vi "Format CSV.vi"(8 "error in (no error)":errorcluster, 9 "delimiter":string=",", 10 "CSV File Input":path, 11 "Original CSV Format":enum16{"Format A", "Format B"}(ring)) -> (0 "error out":errorcluster, 1 "Parcel Length":i32[](array[numeric]), 2 "All Terminal Data":T1(array[cluster]))   [LabVIEW 2017] (continued)
"48:51.9", "48:51.9", "48:51.9", "48:52.0", "48:52.0", "48:52.0", "48:52.1", "48:52.1", "48:52.1", "48:52.2", "48:52.2", "48:52.2", "48:52.3", "48:52.3", "48:52.3", "48:52.4", "48:52.4", "48:52.4", "48:52.5", "48:52.5", "48:52.5", "48:52.6", "48:52.6", "48:52.6", "48:52.7", "48:52.7", "48:52.7", "48:52.8", "48:52.8", "48:52.8", "48:52.9", "48:52.9", "48:52.9", "48:53.0", "48:53.0", "48:53.0", "48:53.1", "48:53.1", "48:53.1", "48:53.2", "48:53.2", "48:53.2", "48:53.3", "48:53.3", "48:53.3", "48:53.4", "48:53.4", "48:53.4", "48:53.5", "48:53.5", "48:53.5", "48:53.6", "48:53.6", "48:53.6", "48:53.7", "48:53.7", "48:53.7", "48:53.8", "48:53.8", "48:53.8", "48:53.9", "48:53.9", "48:53.9", "48:54.0", "48:54.0", "48:54.0", "48:54.1", "48:54.1", "48:54.1", "48:54.2", "48:54.2", "48:54.2", "48:54.3", "48:54.3", "48:54.3", "48:54.4", "48:54.4", "48:54.4", "48:54.5", "48:54.5", "48:54.5", "48:54.6", "48:54.6", "48:54.6", "48:54.7", "48:54.7", "48:54.7", "48:54.8", "48:54.8", "48:54.8", "48:54.9", "48:54.9", "48:54.9", "48:55.0", "48:55.0", "48:55.0", "48:55.1", "48:55.1", "48:55.1", "48:55.2", "48:55.2", "48:55.2", "48:55.3", "48:55.3", "48:55.3", "48:55.4", "48:55.4", "48:55.4", "48:55.5", "48:55.5", "48:55.5", "48:55.6", "48:55.6", "48:55.6", "48:55.7", "48:55.7", "48:55.7", "48:55.8", "48:55.8", "48:55.8", "48:55.9", "48:55.9", "48:55.9", "48:56.0", "48:56.0", "48:56.0", "48:56.1", "48:56.1", "48:56.1", "48:56.2", "48:56.2", "48:56.2", "48:56.3", "48:56.3", "48:56.3", "48:56.4", "48:56.4", "48:56.4", "48:56.5", "48:56.5", "48:56.5", "48:56.6", "48:56.6", "48:56.6", "48:56.7", "48:56.7", "48:56.7", "48:56.8", "48:56.8", "48:56.8", "48:56.9", "48:56.9", "48:56.9", "48:57.0", "48:57.0", "48:57.0", "48:57.1", "48:57.1", "48:57.1", "48:57.2", "48:57.2", "48:57.2", "48:57.3", "48:57.3", "48:57.3", "48:57.4", "48:57.4", "48:57.4", "48:57.5", "48:57.5", "48:57.5", "48:57.6", "48:57.6", "48:57.6", "48:57.7", "48:57.7", "48:57.7", "48:57.8", "48:57.8", "48:57.8", "48:57.9", "48:57.9", "48:57.9", "48:58.0", "48:58.0", "48:58.0", "48:58.1", "48:58.1", "48:58.1", "48:58.2", "48:58.2", "48:58.2", "48:58.3", "48:58.3", "48:58.3", "48:58.4", "48:58.4", "48:58.4", "48:58.5", "48:58.5", "48:58.5", "48:58.6", "48:58.6", "48:58.6", "48:58.7", "48:58.7", "48:58.7", "48:58.8", "48:58.8", "48:58.8", "48:58.9", "48:58.9", "48:58.9", "48:59.0", "48:59.0", "48:59.0", "48:59.1", "48:59.1", "48:59.1", "48:59.2", "48:59.2", "48:59.2", "48:59.3", "48:59.3", "48:59.3", "48:59.4", "48:59.4", "48:59.4", "48:59.5", "48:59.5", "48:59.5", "48:59.6", "48:59.6", "48:59.6", "48:59.7", "48:59.7", "48:59.7", "48:59.8", "48:59.8", "48:59.8", "48:59.9", "48:59.9", "48:59.9", "49:00.0", "49:00.0", "49:00.0", "49:00.1", "49:00.1", "49:00.1", "49:00.2", "49:00.2", "49:00.2", "49:00.3", "49:00.3", "49:00.3", "49:00.4", "49:00.4", "49:00.4", "49:00.5", "49:00.5", "49:00.5", "49:00.6", "49:00.6", "49:00.6", "49:00.7", "49:00.7", "49:00.7", "49:00.8", "49:00.8", "49:00.8", "49:00.9", "49:00.9", "49:00.9", "49:01.0", "49:01.0", "49:01.0", "49:01.1", "49:01.1", "49:01.1", "49:01.2", "49:01.2", "49:01.2", "49:01.3", "49:01.3", "49:01.3", "49:01.4", "49:01.4", "49:01.4", "49:01.5", "49:01.5", "49:01.5", "49:01.6", "49:01.6", "49:01.6", "49:01.7", "49:01.7", "49:01.7", "49:01.8", "49:01.8", "49:01.8", "49:01.9", "49:01.9", "49:01.9", "49:02.0", "49:02.0", "49:02.0", "49:02.1", "49:02.1", "49:02.1", "49:02.2", "49:02.2", "49:02.2", "49:02.3", "49:02.3", "49:02.3", "49:02.4", "49:02.4", "49:02.4", "49:02.5", "49:02.5", "49:02.5", "49:02.6", "49:02.6", "49:02.6", "49:02.7", "49:02.7", "49:02.7", "49:02.8", "49:02.8", "49:02.8", "49:02.9", "49:02.9", "49:02.9", "49:03.0", "49:03.0", "49:03.0", "49:03.1", "49:03.1", "49:03.1", "49:03.2", "49:03.2", "49:03.2", "49:03.3", "49:03.3", "49:03.3", "49:03.4", "49:03.4", "49:03.4", "49:03.5", "49:03.5", "49:03.5", "49:03.6", "49:03.6", "49:03.6", "49:03.7", "49:03.7", "49:03.7", "49:03.8", "49:03.8", "49:03.8", "49:03.9", "49:03.9", "49:03.9", "49:04.0", "49:04.0", "49:04.0", "49:04.1", "49:04.1", "49:04.1", "49:04.2", "49:04.2", "49:04.2", "49:04.3", "49:04.3", "49:04.3", "49:04.4", "49:04.4", "49:04.4", "49:04.5", "49:04.5", "49:04.5", "49:04.6", "49:04.6", "49:04.6", "49:04.7", "49:04.7", "49:04.7", "49:04.8", "49:04.8", "49:04.8", "49:04.9", "49:04.9", "49:04.9", "49:05.0", "49:05.0", "49:05.0", "49:05.1", "49:05.1", "49:05.1", "49:05.2", "49:05.2", "49:05.2", "49:05.3", "49:05.3", "49:05.3", "49:05.4", "49:05.4", "49:05.4", "49:05.5", "49:05.5", "49:05.5", "49:05.6", "49:05.6", "49:05.6", "49:05.7", "49:05.7", "49:05.7", "49:05.8", "49:05.8", "49:05.8", "49:05.9", "49:05.9", "49:05.9", "49:06.0", "49:06.0", "49:06.0", "49:06.1", "49:06.1", "49:06.1", "49:06.2", "49:06.2", "49:06.2", "49:06.3", "49:06.3", "49:06.3", "49:06.4", "49:06.4", "49:06.4", "49:06.5", "49:06.5", "49:06.5", "49:06.6", "49:06.6", "49:06.6", "49:06.7", "49:06.7", "49:06.7", "49:06.8", "49:06.8", "49:06.8", "49:06.9", "49:06.9", "49:06.9", "49:07.0", "49:07.0", "49:07.0", "49:07.1", "49:07.1", "49:07.1", "49:07.2", "49:07.2", "49:07.2", "49:07.3", "49:07.3", "49:07.3", "49:07.4", "49:07.4", "49:07.4", "49:07.5", "49:07.5", "49:07.5", "49:07.6", "49:07.6", "49:07.6", "49:07.7", "49:07.7", "49:07.7", "49:07.8", "49:07.8", "49:07.8", "49:07.9", "49:07.9", "49:07.9", "49:08.0", "49:08.0", "49:08.0", "49:08.1", "49:08.1", "49:08.1", "49:08.2", "49:08.2", "49:08.2", "49:08.3", "49:08.3", "49:08.3", "49:08.4", "49:08.4", "49:08.4", "49:08.5", "49:08.5", "49:08.5", "49:08.6", "49:08.6", "49:08.6", "49:08.7", "49:08.7", "49:08.7", "49:08.8", "49:08.8", "49:08.8", "49:08.9", "49:08.9", "49:08.9", "49:09.0", "49:09.0", "49:09.0", "49:09.1", "49:09.1", "49:09.1", "49:09.2", "49:09.2", "49:09.2", "49:09.3", "49:09.3", "49:09.3", "49:09.4", "49:09.4", "49:09.4", "49:09.5", "49:09.5", "49:09.5", "49:09.6", "49:09.6", "49:09.6", "49:09.7", "49:09.7", "49:09.7", "49:09.8", "49:09.8", "49:09.8", "49:09.9", "49:09.9", "49:09.9", "49:10.0", "49:10.0", "49:10.0", "49:10.1", "49:10.1", "49:10.1", "49:10.2", "49:10.2", "49:10.2", "49:10.3", "49:10.3", "49:10.3", "49:10.4", "49:10.4", "49:10.4", "49:10.5", "49:10.5", "49:10.5", "49:10.6", "49:10.6", "49:10.6", "49:10.7", "49:10.7", "49:10.7", "49:10.8", "49:10.8", "49:10.8", "49:10.9", "49:10.9", "49:10.9", "49:11.0", "49:11.0", "49:11.0", "49:11.1", "49:11.1", "49:11.1", "49:11.2", "49:11.2", "49:11.2", "49:11.3", "49:11.3", "49:11.3", "49:11.4", "49:11.4", "49:11.4", "49:11.5", "49:11.5", "49:11.5", "49:11.6", "49:11.6", "49:11.6", "49:11.7", "49:11.7", "49:11.7", "49:11.8", "49:11.8", "49:11.8", "49:11.9", "49:11.9", "49:11.9", "49:12.0", "49:12.0", "49:12.0", "49:12.1", "49:12.1", "49:12.1", "49:12.2", "49:12.2", "49:12.2", "49:12.3", "49:12.3", "49:12.3", "49:12.4", "49:12.4", "49:12.4", "49:12.5", "49:12.5", "49:12.5", "49:12.6", "49:12.6", "49:12.6", "49:12.7", "49:12.7", "49:12.7", "49:12.8", "49:12.8", "49:12.8", "49:12.9", "49:12.9", "49:12.9", "49:13.0", "49:13.0", "49:13.0", "49:13.1", "49:13.1", "49:13.1", "49:13.2", "49:13.2", "49:13.2", "49:13.3", "49:13.3", "49:13.3", "49:13.4", "49:13.4", "49:13.4", "49:13.5", "49:13.5", "49:13.5", "49:13.6", "49:13.6", "49:13.6", "49:13.7", "49:13.7", "49:13.7", "49:13.8", "49:13.8", "49:13.8", "49:13.9", "49:13.9", "49:13.9", "49:14.0", "49:14.0", "49:14.0", "49:14.1", "49:14.1", "49:14.1", "49:14.2", "49:14.2", "49:14.2", "49:14.3", "49:14.3", "49:14.3", "49:14.4", "49:14.4", "49:14.4", "49:14.5", "49:14.5", "49:14.5", "49:14.6", "49:14.6", "49:14.6", "49:14.7", "49:14.7", "49:14.7", "49:14.8", "49:14.8", "49:14.8", "49:14.9", "49:14.9", "49:14.9", "49:15.0", "49:15.0", "49:15.0", "49:15.1", "49:15.1", "49:15.1", "49:15.2", "49:15.2", "49:15.2", "49:15.3", "49:15.3", "49:15.3", "49:15.4", "49:15.4", "49:15.4", "49:15.5", "49:15.5", "49:15.5", "49:15.6", "49:15.6", "49:15.6", "49:15.7", "49:15.7", "49:15.7", "49:15.8", "49:15.8", "49:15.8", "49:15.9", "49:15.9", "49:15.9", "49:16.0", "49:16.0", "49:16.0", "49:16.1", "49:16.1", "49:16.1", "49:16.2", "49:16.2", "49:16.2", "49:16.3", "49:16.3", "49:16.3", "49:16.4", "49:16.4", "49:16.4", "49:16.5", "49:16.5", "49:16.5", "49:16.6", "49:16.6", "49:16.6", "49:16.7", "49:16.7", "49:16.7", "49:16.8", "49:16.8", "49:16.8", "49:16.9", "49:16.9", "49:16.9", "49:17.0", "49:17.0", "49:17.0", "49:17.1", "49:17.1", "49:17.1", "49:17.2", "49:17.2", "49:17.2", "49:17.3", "49:17.3", "49:17.3", "49:17.4", "49:17.4", "49:17.4", "49:17.5", "49:17.5", "49:17.5", "49:17.6", "49:17.6", "49:17.6", "49:17.7", "49:17.7", "49:17.7", "49:17.8", "49:17.8", "49:17.8", "49:17.9", "49:17.9", "49:17.9", "49:18.0", "49:18.0", "49:18.0", "49:18.1", "49:18.1", "49:18.1", "49:18.2", "49:18.2", "49:18.2", "49:18.3", "49:18.3", "49:18.3", "49:18.4", "49:18.4", "49:18.4", "49:18.5", "49:18.5", "49:18.5", "49:18.6", "49:18.6", "49:18.6", "49:18.7", "49:18.7", "49:18.7", "49:18.8", "49:18.8", "49:18.8", "49:18.9", "49:18.9", "49:18.9", "49:19.0", "49:19.0", "49:19.0", "49:19.1", "49:19.1", "49:19.1", "49:19.2", "49:19.2", "49:19.2", "49:19.3", "49:19.3", "49:19.3", "49:19.4", "49:19.4", "49:19.4", "49:19.5", "49:19.5", "49:19.5", "49:19.6", "49:19.6", "49:19.6", "49:19.7", "49:19.7", "49:19.7", "49:19.8", "49:19.8", "49:19.8", "49:19.9", "49:19.9", "49:19.9", "49:20.0", "49:20.0", "49:20.0", "49:20.1", "49:20.1", "49:20.1", "49:20.2", "49:20.2", "49:20.2", "49:20.3", "49:20.3", "49:20.3", "49:20.4", "49:20.4", "49:20.4", "49:20.5", "49:20.5", "49:20.5", "49:20.6", "49:20.6", "49:20.6", "49:20.7", "49:20.7", "49:20.7", "49:20.8", "49:20.8", "49:20.8", "49:20.9", "49:20.9", "49:20.9", "49:21.0", "49:21.0", "49:21.0", "49:21.1", "49:21.1", "49:21.1", "49:21.2", "49:21.2", "49:21.2", "49:21.3", "49:21.3", "49:21.3", "49:21.4", "49:21.4", "49:21.4", "49:21.5", "49:21.5", "49:21.5", "49:21.6", "49:21.6", "49:21.6", "49:21.7", "49:21.7", "49:21.7", "49:21.8", "49:21.8", "49:21.8", "49:21.9", "49:21.9", "49:21.9", "49:22.0", "49:22.0", "49:22.0", "49:22.1", "49:22.1", "49:22.1", "49:22.2", "49:22.2", "49:22.2", "49:22.3", "49:22.3", "49:22.3", "49:22.4", "49:22.4", "49:22.4", "49:22.5", "49:22.5", "49:22.5", "49:22.6", "49:22.6", "49:22.6", "49:22.7", "49:22.7", "49:22.7", "49:22.8", "49:22.8", "49:22.8", "49:22.9", "49:22.9", "49:22.9", "49:23.0", "49:23.0", "49:23.0", "49:23.1", "49:23.1", "49:23.1", "49:23.2", "49:23.2", "49:23.2", "49:23.3", "49:23.3", "49:23.3", "49:23.4", "49:23.4", "49:23.4", "49:23.5", "49:23.5", "49:23.5", "49:23.6", "49:23.6", "49:23.6", "49:23.7", "49:23.7", "49:23.7", "49:23.8", "49:23.8", "49:23.8", "49:23.9", "49:23.9", "49:23.9", "49:24.0", "49:24.0", "49:24.0", "49:24.1", "49:24.1", "49:24.1", "49:24.2", "49:24.2", "49:24.2", "49:24.3", "49:24.3", "49:24.3", "49:24.4", "49:24.4", "49:24.4", "49:24.5", "49:24.5", "49:24.5", "49:24.6", "49:24.6", "49:24.6", "49:24.7", "49:24.7", "49:24.7", "49:24.8", "49:24.8", "49:24.8", "49:24.9", "49:24.9", "49:24.9", "49:25.0", "49:25.0", "49:25.0", "49:25.1", "49:25.1", "49:25.1", "49:25.2", "49:25.2", "49:25.2", "49:25.3", "49:25.3", "49:25.3", "49:25.4", "49:25.4", "49:25.4", "49:25.5", "49:25.5", "49:25.5", "49:25.6", "49:25.6", "49:25.6", "49:25.7", "49:25.7", "49:25.7", "49:25.8", "49:25.8", "49:25.8", "49:25.9", "49:25.9", "49:25.9", "49:26.0", "49:26.0", "49:26.0", "49:26.1", "49:26.1", "49:26.1", "49:26.2", "49:26.2", "49:26.2", "49:26.3", "49:26.3", "49:26.3", "49:26.4", "49:26.4", "49:26.4", "49:26.5", "49:26.5", "49:26.5", "49:26.6", "49:26.6", "49:26.6", "49:26.7", "49:26.7", "49:26.7", "49:26.8", "49:26.8", "49:26.8", "49:26.9", "49:26.9", "49:26.9", "49:27.0", "49:27.0", "49:27.0", "49:27.1", "49:27.1", "49:27.1", "49:27.2", "49:27.2", "49:27.2", "49:27.3", "49:27.3", "49:27.3", "49:27.4", "49:27.4", "49:27.4", "49:27.5", "49:27.5", "49:27.5", "49:27.6", "49:27.6", "49:27.6", "49:27.7", "49:27.7", "49:27.7", "49:27.8", "49:27.8", "49:27.8", "49:27.9", "49:27.9", "49:27.9", "49:28.0", "49:28.0", "49:28.0", "49:28.1", "49:28.1", "49:28.1", "49:28.2", "49:28.2", "49:28.2", "49:28.3", "49:28.3", "49:28.3", "49:28.4", "49:28.4", "49:28.4", "49:28.5", "49:28.5", "49:28.5", "49:28.6", "49:28.6", "49:28.6", "49:28.7", "49:28.7", "49:28.7", "49:28.8", "49:28.8", "49:28.8", "49:28.9", "49:28.9", "49:28.9", "49:29.0", "49:29.0", "49:29.0", "49:29.1", "49:29.1", "49:29.1", "49:29.2", "49:29.2", "49:29.2", "49:29.3", "49:29.3", "49:29.3", "49:29.4", "49:29.4", "49:29.4", "49:29.5", "49:29.5", "49:29.5", "49:29.6", "49:29.6", "49:29.6", "49:29.7", "49:29.7", "49:29.7", "49:29.8", "49:29.8", "49:29.8", "49:29.9", "49:29.9", "49:29.9", "49:30.0", "49:30.0", "49:30.0", "49:30.1", "49:30.1", "49:30.1", "49:30.2", "49:30.2", "49:30.2", "49:30.3", "49:30.3", "49:30.3", "49:30.4", "49:30.4", "49:30.4", "49:30.5", "49:30.5", "49:30.5", "49:30.6", "49:30.6", "49:30.6", "49:30.7", "49:30.7", "49:30.7", "49:30.8", "49:30.8", "49:30.8", "49:30.9", "49:30.9", "49:30.9", "49:31.0", "49:31.0", "49:31.0", "49:31.1", "49:31.1", "49:31.1", "49:31.2", "49:31.2", "49:31.2", "49:31.3", "49:31.3", "49:31.3", "49:31.4", "49:31.4", "49:31.4", "49:31.5", "49:31.5", "49:31.5", "49:31.6", "49:31.6", "49:31.6", "49:31.7", "49:31.7", "49:31.7", "49:31.8", "49:31.8", "49:31.8", "49:31.9", "49:31.9", "49:31.9", "49:32.0", "49:32.0", "49:32.0", "49:32.1", "49:32.1", "49:32.1", "49:32.2", "49:32.2", "49:32.2", "49:32.3", "49:32.3", "49:32.3", "49:32.4", "49:32.4", "49:32.4", "49:32.5", "49:32.5", "49:32.5", "49:32.6", "49:32.6", "49:32.6", "49:32.7", "49:32.7", "49:32.7", "49:32.8", "49:32.8", "49:32.8", "49:32.9", "49:32.9", "49:32.9", "49:33.0", "49:33.0", "49:33.0", "49:33.1", "49:33.1", "49:33.1", "49:33.2", "49:33.2", "49:33.2", "49:33.3", "49:33.3", "49:33.3", "49:33.4", "49:33.4", "49:33.4", "49:33.5", "49:33.5", "49:33.5", "49:33.6", "49:33.6", "49:33.6", "49:33.7", "49:33.7", "49:33.7", "49:33.8", "49:33.8", "49:33.8", "49:33.9", "49:33.9", "49:33.9", "49:34.0", "49:34.0", "49:34.0", "49:34.1", "49:34.1", "49:34.1", "49:34.2", "49:34.2", "49:34.2", "49:34.3", "49:34.3", "49:34.3", "49:34.4", "49:34.4", "49:34.4", "49:34.5", "49:34.5", "49:34.5", "49:34.6", "49:34.6", "49:34.6", "49:34.7", "49:34.7", "49:34.7", "49:34.8", "49:34.8", "49:34.8", "49:34.9", "49:34.9", "49:34.9", "49:35.0", "49:35.0", "49:35.0", "49:35.1", "49:35.1", "49:35.1", "49:35.2", "49:35.2", "49:35.2", "49:35.3", "49:35.3", "49:35.3", "49:35.4", "49:35.4", "49:35.4", "49:35.5", "49:35.5", "49:35.5", "49:35.6", "49:35.6", "49:35.6", "49:35.7", "49:35.7", "49:35.7", "49:35.8", "49:35.8", "49:35.8", "49:35.9", "49:35.9", "49:35.9", "49:36.0", "49:36.0", "49:36.0", "49:36.1", "49:36.1", "49:36.1", "49:36.2", "49:36.2", "49:36.2", "49:36.3", "49:36.3", "49:36.3", "49:36.4", "49:36.4", "49:36.4", "49:36.5", "49:36.5", "49:36.5", "49:36.6", "49:36.6", "49:36.6", "49:36.7", "49:36.7", "49:36.7", "49:36.8", "49:36.8", "49:36.8", "49:36.9", "49:36.9", "49:36.9", "49:37.0", "49:37.0", "49:37.0", "49:37.1", "49:37.1", "49:37.1", "49:37.2", "49:37.2", "49:37.2", "49:37.3", "49:37.3", "49:37.3", "49:37.4", "49:37.4", "49:37.4", "49:37.5", "49:37.5", "49:37.5", "49:37.6", "49:37.6", "49:37.6", "49:37.7", "49:37.7", "49:37.7", "49:37.8", "49:37.8", "49:37.8", "49:37.9", "49:37.9", "49:37.9", "49:38.0", "49:38.0", "49:38.0", "49:38.1", "49:38.1", "49:38.1", "49:38.2", "49:38.2", "49:38.2", "49:38.3", "49:38.3", "49:38.3", "49:38.4", "49:38.4", "49:38.4", "49:38.5", "49:38.5", "49:38.5", "49:38.6", "49:38.6", "49:38.6", "49:38.7", "49:38.7", "49:38.7", "49:38.8", "49:38.8", "49:38.8", "49:38.9", "49:38.9", "49:38.9", "49:39.0", "49:39.0", "49:39.0", "49:39.1", "49:39.1", "49:39.1", "49:39.2", "49:39.2", "49:39.2", "49:39.3", "49:39.3", "49:39.3", "49:39.4", "49:39.4", "49:39.4", "49:39.5", "49:39.5", "49:39.5", "49:39.6", "49:39.6", "49:39.6", "49:39.7", "49:39.7", "49:39.7", "49:39.8", "49:39.8", "49:39.8", "49:39.9", "49:39.9", "49:39.9", "49:40.0", "49:40.0", "49:40.0", "49:40.1", "49:40.1", "49:40.1", "49:40.2", "49:40.2", "49:40.2", "49:40.3", "49:40.3", "49:40.3", "49:40.4", "49:40.4", "49:40.4", "49:40.5", "49:40.5", "49:40.5", "49:40.6", "49:40.6", "49:40.6", "49:40.7", "49:40.7", "49:40.7", "49:40.8", "49:40.8", "49:40.8", "49:40.9", "49:40.9", "49:40.9", "49:41.0", "49:41.0", "49:41.0", "49:41.1", "49:41.1", "49:41.1", "49:41.2", "49:41.2", "49:41.2", "49:41.3", "49:41.3", "49:41.3", "49:41.4", "49:41.4", "49:41.4", "49:41.5", "49:41.5", "49:41.5", "49:41.6", "49:41.6", "49:41.6", "49:41.7", "49:41.7", "49:41.7", "49:41.8", "49:41.8", "49:41.8", "49:41.9", "49:41.9", "49:41.9", "49:42.0", "49:42.0", "49:42.0", "49:42.1", "49:42.1", "49:42.1", "49:42.2", "49:42.2", "49:42.2", "49:42.3", "49:42.3", "49:42.3", "49:42.4", "49:42.4", "49:42.4", "49:42.5", "49:42.5", "49:42.5", "49:42.6", "49:42.6", "49:42.6", "49:42.7", "49:42.7", "49:42.7", "49:42.8", "49:42.8", "49:42.8", "49:42.9", "49:42.9", "49:42.9", "49:43.0", "49:43.0", "49:43.0", "49:43.1", "49:43.1", "49:43.1", "49:43.2", "49:43.2", "49:43.2", "49:43.3", "49:43.3", "49:43.3", "49:43.4", "49:43.4", "49:43.4", "49:43.5", "49:43.5", "49:43.5", "49:43.6", "49:43.6", "49:43.6", "49:43.7", "49:43.7", "49:43.7", "49:43.8", "49:43.8", "49:43.8", "49:43.9", "49:43.9", "49:43.9", "49:44.0", "49:44.0", "49:44.0", "49:44.1", "49:44.1", "49:44.1", "49:44.2", "49:44.2", "49:44.2", "49:44.3", "49:44.3", "49:44.3", "49:44.4", "49:44.4", "49:44.4", "49:44.5", "49:44.5", "49:44.5", "49:44.6", "49:44.6", "49:44.6", "49:44.7", "49:44.7", "49:44.7", "49:44.8", "49:44.8", "49:44.8", "49:44.9", "49:44.9", "49:44.9", "49:45.0", "49:45.0", "49:45.0", "49:45.1", "49:45.1", "49:45.1", "49:45.2", "49:45.2", "49:45.2", "49:45.3", "49:45.3", "49:45.3", "49:45.4", "49:45.4", "49:45.4", "49:45.5", "49:45.5", "49:45.5", "49:45.6", "49:45.6", "49:45.6", "49:45.7", "49:45.7", "49:45.7", "49:45.8", "49:45.8", "49:45.8", "49:45.9", "49:45.9", "49:45.9", "49:46.0", "49:46.0", "49:46.0", "49:46.1", "49:46.1", "49:46.1", "49:46.2", "49:46.2", "49:46.2", "49:46.3", "49:46.3", "49:46.3", "49:46.4", "49:46.4", "49:46.4", "49:46.5", "49:46.5", "49:46.5", "49:46.6", "49:46.6", "49:46.6", "49:46.7", "49:46.7", "49:46.7", "49:46.8", "49:46.8", "49:46.8", "49:46.9", "49:46.9", "49:46.9", "49:47.0", "49:47.0", "49:47.0", "49:47.1", "49:47.1", "49:47.1", "49:47.2", "49:47.2", "49:47.2", "49:47.3", "49:47.3", "49:47.3", "49:47.4", "49:47.4", "49:47.4", "49:47.5", "49:47.5", "49:47.5", "49:47.6", "49:47.6", "49:47.6", "49:47.7", "49:47.7", "49:47.7", "49:47.8", "49:47.8", "49:47.8", "49:47.9", "49:47.9", "49:47.9", "49:48.0", "49:48.0", "49:48.0", "49:48.1", "49:48.1", "49:48.1", "49:48.2", "49:48.2", "49:48.2", "49:48.3", "49:48.3", "49:48.3", "49:48.4", "49:48.4", "49:48.4", "49:48.5", "49:48.5", "49:48.5", "49:48.6", "49:48.6", "49:48.6", "49:48.7", "49:48.7", "49:48.7", "49:48.8", "49:48.8", "49:48.8", "49:48.9", "49:48.9", "49:48.9", "49:49.0", "49:49.0", "49:49.0", "49:49.1", "49:49.1", "49:49.1", "49:49.2", "49:49.2", "49:49.2", "49:49.3", "49:49.3", "49:49.3", "49:49.4", "49:49.4", "49:49.4", "49:49.5", "49:49.5", "49:49.5", "49:49.6", "49:49.6", "49:49.6", "49:49.7", "49:49.7", "49:49.7", "49:49.8", "49:49.8", "49:49.8", "49:49.9", "49:49.9", "49:49.9", "49:50.0", "49:50.0", "49:50.0", "49:50.1", "49:50.1", "49:50.1", "49:50.2", "49:50.2", "49:50.2", "49:50.3", "49:50.3", "49:50.3", "49:50.4", "49:50.4", "49:50.4", "49:50.5", "49:50.5", "49:50.5", "49:50.6", "49:50.6", "49:50.6", "49:50.7", "49:50.7", "49:50.7", "49:50.8", "49:50.8", "49:50.8", "49:50.9", "49:50.9", "49:50.9", "49:51.0", "49:51.0", "49:51.0", "49:51.1", "49:51.1", "49:51.1", "49:51.2", "49:51.2", "49:51.2", "49:51.3", "49:51.3", "49:51.3", "49:51.4", "49:51.4", "49:51.4", "49:51.5", "49:51.5", "49:51.5", "49:51.6", "49:51.6", "49:51.6", "49:51.7", "49:51.7", "49:51.7", "49:51.8", "49:51.8", "49:51.8", "49:51.9", "49:51.9", "49:51.9", "49:52.0", "49:52.0", "49:52.0", "49:52.1", "49:52.1", "49:52.1", "49:52.2", "49:52.2", "49:52.2", "49:52.3", "49:52.3", "49:52.3", "49:52.4", "49:52.4", "49:52.4", "49:52.5", "49:52.5", "49:52.5", "49:52.6", "49:52.6", "49:52.6", "49:52.7", "49:52.7", "49:52.7", "49:52.8", "49:52.8", "49:52.8", "49:52.9", "49:52.9", "49:52.9", "49:53.0", "49:53.0", "49:53.0", "49:53.1", "49:53.1", "49:53.1", "49:53.2", "49:53.2", "49:53.2", "49:53.3", "49:53.3", "49:53.3", "49:53.4", "49:53.4", "49:53.4", "49:53.5", "49:53.5", "49:53.5", "49:53.6", "49:53.6", "49:53.6", "49:53.7", "49:53.7", "49:53.7", "49:53.8", "49:53.8", "49:53.8", "49:53.9", "49:53.9", "49:53.9", "49:54.0", "49:54.0", "49:54.0", "49:54.1", "49:54.1", "49:54.1", "49:54.2", "49:54.2", "49:54.2", "49:54.3", "49:54.3", "49:54.3", "49:54.4", "49:54.4", "49:54.4", "49:54.5", "49:54.5", "49:54.5", "49:54.6", "49:54.6", "49:54.6", "49:54.7", "49:54.7", "49:54.7", "49:54.8", "49:54.8", "49:54.8", "49:54.9", "49:54.9", "49:54.9", "49:55.0", "49:55.0", "49:55.0", "49:55.1", "49:55.1", "49:55.1", "49:55.2", "49:55.2", "49:55.2", "49:55.3", "49:55.3", "49:55.3", "49:55.4", "49:55.4", "49:55.4", "49:55.5", "49:55.5", "49:55.5", "49:55.6", "49:55.6", "49:55.6", "49:55.7", "49:55.7", "49:55.7", "49:55.8", "49:55.8", "49:55.8", "49:55.9", "49:55.9", "49:55.9", "49:56.0", "49:56.0", "49:56.0", "49:56.1", "49:56.1", "49:56.1", "49:56.2", "49:56.2", "49:56.2", "49:56.3", "49:56.3", "49:56.3", "49:56.4", "49:56.4", "49:56.4", "49:56.5", "49:56.5", "49:56.5", "49:56.6", "49:56.6", "49:56.6", "49:56.7", "49:56.7", "49:56.7", "49:56.8", "49:56.8", "49:56.8", "49:56.9", "49:56.9", "49:56.9", "49:57.0", "49:57.0", "49:57.0", "49:57.1", "49:57.1", "49:57.1", "49:57.2", "49:57.2", "49:57.2", "49:57.3", "49:57.3", "49:57.3", "49:57.4", "49:57.4", "49:57.4", "49:57.5", "49:57.5", "49:57.5", "49:57.6", "49:57.6", "49:57.6", "49:57.7", "49:57.7", "49:57.7", "49:57.8", "49:57.8", "49:57.8", "49:57.9", "49:57.9", "49:57.9", "49:58.0", "49:58.0", "49:58.0", "49:58.1", "49:58.1", "49:58.1", "49:58.2", "49:58.2", "49:58.2", "49:58.3", "49:58.3", "49:58.3", "49:58.4", "49:58.4", "49:58.4", "49:58.5", "49:58.5", "49:58.5", "49:58.6", "49:58.6", "49:58.6", "49:58.7", "49:58.7", "49:58.7", "49:58.8", "49:58.8", "49:58.8", "49:58.9", "49:58.9", "49:58.9", "49:59.0", "49:59.0", "49:59.0", "49:59.1", "49:59.1", "49:59.1", "49:59.2", "49:59.2", "49:59.2", "49:59.3", "49:59.3", "49:59.3", "49:59.4", "49:59.4", "49:59.4", "49:59.5", "49:59.5", "49:59.5", "49:59.6", "49:59.6", "49:59.6", "49:59.7", "49:59.7", "49:59.7", "49:59.8", "49:59.8", "49:59.8", "49:59.9", "49:59.9", "49:59.9", "50:00.0", "50:00.0", "50:00.0", "50:00.1", "50:00.1", "50:00.1", "50:00.2", "50:00.2", "50:00.2", "50:00.3", "50:00.3", "50:00.3", "50:00.4", "50:00.4", "50:00.4", "50:00.5", "50:00.5", "50:00.5", "50:00.6", "50:00.6", "50:00.6", "50:00.7", "50:00.7", "50:00.7", "50:00.8", "50:00.8", "50:00.8", "50:00.9", "50:00.9", "50:00.9", "50:01.0", "50:01.0", "50:01.0", "50:01.1", "50:01.1", "50:01.1", "50:01.2", "50:01.2", "50:01.2", "50:01.3", "50:01.3", "50:01.3", "50:01.4", "50:01.4", "50:01.4", "50:01.5", "50:01.5", "50:01.5", "50:01.6", "50:01.6", "50:01.6", "50:01.7", "50:01.7", "50:01.7", "50:01.8", "50:01.8", "50:01.8", "50:01.9", "50:01.9", "50:01.9", "50:02.0", "50:02.0", "50:02.0", "50:02.1", "50:02.1", "50:02.1", "50:02.2", "50:02.2", "50:02.2", "50:02.3", "50:02.3", "50:02.3", "50:02.4", "50:02.4", "50:02.4", "50:02.5", "50:02.5", "50:02.5", "50:02.6", "50:02.6", "50:02.6", "50:02.7", "50:02.7", "50:02.7", "50:02.8", "50:02.8", "50:02.8", "50:02.9", "50:02.9", "50:02.9", "50:03.0", "50:03.0", "50:03.0", "50:03.1", "50:03.1", "50:03.1", "50:03.2", "50:03.2", "50:03.2", "50:03.3", "50:03.3", "50:03.3", "50:03.4", "50:03.4", "50:03.4", "50:03.5", "50:03.5", "50:03.5", "50:03.6", "50:03.6", "50:03.6", "50:03.7", "50:03.7", "50:03.7", "50:03.8", "50:03.8", "50:03.8", "50:03.9", "50:03.9", "50:03.9", "50:04.0", "50:04.0", "50:04.0", "50:04.1", "50:04.1", "50:04.1", "50:04.2", "50:04.2", "50:04.2", "50:04.3", "50:04.3", "50:04.3", "50:04.4", "50:04.4", "50:04.4", "50:04.5", "50:04.5", "50:04.5", "50:04.6", "50:04.6", "50:04.6", "50:04.7", "50:04.7", "50:04.7", "50:04.8", "50:04.8", "50:04.8", "50:04.9", "50:04.9", "50:04.9", "50:05.0", "50:05.0", "50:05.0", "50:05.1", "50:05.1", "50:05.1", "50:05.2", "50:05.2", "50:05.2", "50:05.3", "50:05.3", "50:05.3", "50:05.4", "50:05.4", "50:05.4", "50:05.5", "50:05.5", "50:05.5", "50:05.6", "50:05.6", "50:05.6", "50:05.7", "50:05.7", "50:05.7", "50:05.8", "50:05.8", "50:05.8", "50:05.9", "50:05.9", "50:05.9", "50:06.0", "50:06.0", "50:06.0", "50:06.1", "50:06.1", "50:06.1", "50:06.2", "50:06.2", "50:06.2", "50:06.3", "50:06.3", "50:06.3", "50:06.4", "50:06.4", "50:06.4", "50:06.5", "50:06.5", "50:06.5", "50:06.6", "50:06.6", "50:06.6", "50:06.7", "50:06.7", "50:06.7", "50:06.8", "50:06.8", "50:06.8", "50:06.9", "50:06.9", "50:06.9", "50:07.0", "50:07.0", "50:07.0", "50:07.1", "50:07.1", "50:07.1", "50:07.2", "50:07.2", "50:07.2", "50:07.3", "50:07.3", "50:07.3", "50:07.4", "50:07.4", "50:07.4", "50:07.5", "50:07.5", "50:07.5", "50:07.6", "50:07.6", "50:07.6", "50:07.7", "50:07.7", "50:07.7", "50:07.8", "50:07.8", "50:07.8", "50:07.9", "50:07.9", "50:07.9", "50:08.0", "50:08.0", "50:08.0", "50:08.1", "50:08.1", "50:08.1", "50:08.2", "50:08.2", "50:08.2", "50:08.3", "50:08.3", "50:08.3", "50:08.4", "50:08.4", "50:08.4", "50:08.5", "50:08.5", "50:08.5", "50:08.6", "50:08.6", "50:08.6", "50:08.7", "50:08.7", "50:08.7", "50:08.8", "50:08.8", "50:08.8", "50:08.9", "50:08.9", "50:08.9", "50:09.0", "50:09.0", "50:09.0", "50:09.1", "50:09.1", "50:09.1", "50:09.2", "50:09.2", "50:09.2", "50:09.3", "50:09.3", "50:09.3", "50:09.4", "50:09.4", "50:09.4", "50:09.5", "50:09.5", "50:09.5", "50:09.6", "50:09.6", "50:09.6", "50:09.7", "50:09.7", "50:09.7", "50:09.8", "50:09.8", "50:09.8", "50:09.9", "50:09.9", "50:09.9", "50:10.0", "50:10.0", "50:10.0", "50:10.1", "50:10.1", "50:10.1", "50:10.2", "50:10.2", "50:10.2", "50:10.3", "50:10.3", "50:10.3", "50:10.4", "50:10.4", "50:10.4", "50:10.5", "50:10.5", "50:10.5", "50:10.6", "50:10.6", "50:10.6", "50:10.7", "50:10.7", "50:10.7", "50:10.8", "50:10.8", "50:10.8", "50:10.9", "50:10.9", "50:10.9", "50:11.0", "50:11.0", "50:11.0", "50:11.1", "50:11.1", "50:11.1", "50:11.2", "50:11.2", "50:11.2", "50:11.3", "50:11.3", "50:11.3", "50:11.4", "50:11.4", "50:11.4", "50:11.5", "50:11.5", "50:11.5", "50:11.6", "50:11.6", "50:11.6", "50:11.7", "50:11.7", "50:11.7", "50:11.8", "50:11.8", "50:11.8", "50:11.9", "50:11.9", "50:11.9", "50:12.0", "50:12.0", "50:12.0", "50:12.1", "50:12.1", "50:12.1", "50:12.2", "50:12.2", "50:12.2", "50:12.3", "50:12.3", "50:12.3", "50:12.4", "50:12.4", "50:12.4", "50:12.5", "50:12.5", "50:12.5", "50:12.6", "50:12.6", "50:12.6", "50:12.7", "50:12.7", "50:12.7", "50:12.8", "50:12.8", "50:12.8", "50:12.9", "50:12.9", "50:12.9", "50:13.0", "50:13.0", "50:13.0", "50:13.1", "50:13.1", "50:13.1", "50:13.2", "50:13.2", "50:13.2", "50:13.3", "50:13.3", "50:13.3", "50:13.4", "50:13.4", "50:13.4", "50:13.5", "50:13.5", "50:13.5", "50:13.6", "50:13.6", "50:13.6", "50:13.7", "50:13.7", "50:13.7", "50:13.8", "50:13.8", "50:13.8", "50:13.9", "50:13.9", "50:13.9", "50:14.0", "50:14.0", "50:14.0", "50:14.1", "50:14.1", "50:14.1", "50:14.2", "50:14.2", "50:14.2", "50:14.3", "50:14.3", "50:14.3", "50:14.4", "50:14.4", "50:14.4", "50:14.5", "50:14.5", "50:14.5", "50:14.6", "50:14.6", "50:14.6", "50:14.7", "50:14.7", "50:14.7", "50:14.8", "50:14.8", "50:14.8", "50:14.9", "50:14.9", "50:14.9", "50:15.0", "50:15.0", "50:15.0", "50:15.1", "50:15.1", "50:15.1", "50:15.2", "50:15.2", "50:15.2", "50:15.3", "50:15.3", "50:15.3", "50:15.4", "50:15.4", "50:15.4", "50:15.5", "50:15.5", "50:15.5", "50:15.6", "50:15.6", "50:15.6", "50:15.7", "50:15.7", "50:15.7", "50:15.8", "50:15.8", "50:15.8", "50:15.9", "50:15.9", "50:15.9", "50:16.0", "50:16.0", "50:16.0", "50:16.1", "50:16.1", "50:16.1", "50:16.2", "50:16.2", "50:16.2", "50:16.3", "50:16.3", "50:16.3", "50:16.4", "50:16.4", "50:16.4", "50:16.5", "50:16.5", "50:16.5", "50:16.6", "50:16.6", "50:16.6", "50:16.7", "50:16.7", "50:16.7", "50:16.8", "50:16.8", "50:16.8", "50:16.9", "50:16.9", "50:16.9", "50:17.0", "50:17.0", "50:17.0", "50:17.1", "50:17.1", "50:17.1", "50:17.2", "50:17.2", "50:17.2", "50:17.3", "50:17.3", "50:17.3", "50:17.4", "50:17.4", "50:17.4", "50:17.5", "50:17.5", "50:17.5", "50:17.6", "50:17.6", "50:17.6", "50:17.7", "50:17.7", "50:17.7", "50:17.8", "50:17.8", "50:17.8", "50:17.9", "50:17.9", "50:17.9", "50:18.0", "50:18.0", "50:18.0", "50:18.1", "50:18.1", "50:18.1", "50:18.2", "50:18.2", "50:18.2", "50:18.3", "50:18.3", "50:18.3", "50:18.4", "50:18.4", "50:18.4", "50:18.5", "50:18.5", "50:18.5", "50:18.6", "50:18.6", "50:18.6", "50:18.7", "50:18.7", "50:18.7", "50:18.8", "50:18.8", "50:18.8", "50:18.9", "50:18.9", "50:18.9", "50:19.0", "50:19.0", "50:19.0", "50:19.1", "50:19.1", "50:19.1", "50:19.2", "50:19.2", "50:19.2", "50:19.3", "50:19.3", "50:19.3", "50:19.4", "50:19.4", "50:19.4", "50:19.5", "50:19.5", "50:19.5", "50:19.6", "50:19.6", "50:19.6", "50:19.7", "50:19.7", "50:19.7", "50:19.8", "50:19.8", "50:19.8", "50:19.9", "50:19.9", "50:19.9", "50:20.0", "50:20.0", "50:20.0", "50:20.1", "50:20.1", "50:20.1", "50:20.2", "50:20.2", "50:20.2", "50:20.3", "50:20.3", "50:20.3", "50:20.4", "50:20.4", "50:20.4", "50:20.5", "50:20.5", "50:20.5", "50:20.6", "50:20.6", "50:20.6", "50:20.7", "50:20.7", "50:20.7", "50:20.8", "50:20.8", "50:20.8", "50:20.9", "50:20.9", "50:20.9", "50:21.0", "50:21.0", "50:21.0", "50:21.1", "50:21.1", "50:21.1", "50:21.2", "50:21.2", "50:21.2", "50:21.3", "50:21.3", "50:21.3", "50:21.4", "50:21.4", "50:21.4", "50:21.5", "50:21.5", "50:21.5", "50:21.6", "50:21.6", "50:21.6", "50:21.7", "50:21.7", "50:21.7", "50:21.8", "50:21.8", "50:21.8", "50:21.9", "50:21.9", "50:21.9", "50:22.0", "50:22.0", "50:22.0", "50:22.1", "50:22.1", "50:22.1", "50:22.2", "50:22.2", "50:22.2", "50:22.3", "50:22.3", "50:22.3", "50:22.4", "50:22.4", "50:22.4", "50:22.5", "50:22.5", "50:22.5", "50:22.6", "50:22.6", "50:22.6", "50:22.7", "50:22.7", "50:22.7", "50:22.8", "50:22.8", "50:22.8", "50:22.9", "50:22.9", "50:22.9", "50:23.0", "50:23.0", "50:23.0", "50:23.1", "50:23.1", "50:23.1", "50:23.2", "50:23.2", "50:23.2", "50:23.3", "50:23.3", "50:23.3", "50:23.4", "50:23.4", "50:23.4", "50:23.5", "50:23.5", "50:23.5", "50:23.6", "50:23.6", "50:23.6", "50:23.7", "50:23.7", "50:23.7", "50:23.8", "50:23.8", "50:23.8", "50:23.9", "50:23.9", "50:23.9", "50:24.0", "50:24.0", "50:24.0", "50:24.1", "50:24.1", "50:24.1", "50:24.2", "50:24.2", "50:24.2", "50:24.3", "50:24.3", "50:24.3", "50:24.4", "50:24.4", "50:24.4", "50:24.5", "50:24.5", "50:24.5", "50:24.6", "50:24.6", "50:24.6", "50:24.7", "50:24.7", "50:24.7", "50:24.8", "50:24.8", "50:24.8", "50:24.9", "50:24.9", "50:24.9", "50:25.0", "50:25.0", "50:25.0", "50:25.1", "50:25.1", "50:25.1", "50:25.2", "50:25.2", "50:25.2", "50:25.3", "50:25.3", "50:25.3", "50:25.4", "50:25.4", "50:25.4", "50:25.5", "50:25.5", "50:25.5", "50:25.6", "50:25.6", "50:25.6", "50:25.7", "50:25.7", "50:25.7", "50:25.8", "50:25.8", "50:25.8", "50:25.9", "50:25.9", "50:25.9", "50:26.0", "50:26.0", "50:26.0", "50:26.1", "50:26.1", "50:26.1", "50:26.2", "50:26.2", "50:26.2", "50:26.3", "50:26.3", "50:26.3", "50:26.4", "50:26.4", "50:26.4", "50:26.5", "50:26.5", "50:26.5", "50:26.6", "50:26.6", "50:26.6", "50:26.7", "50:26.7", "50:26.7", "50:26.8", "50:26.8", "50:26.8", "50:26.9", "50:26.9", "50:26.9", "50:27.0", "50:27.0", "50:27.0", "50:27.1", "50:27.1", "50:27.1", "50:27.2", "50:27.2", "50:27.2", "50:27.3", "50:27.3", "50:27.3", "50:27.4", "50:27.4", "50:27.4", "50:27.5", "50:27.5", "50:27.5", "50:27.6", "50:27.6", "50:27.6", "50:27.7", "50:27.7", "50:27.7", "50:27.8", "50:27.8", "50:27.8", "50:27.9", "50:27.9", "50:27.9", "50:28.0", "50:28.0", "50:28.0", "50:28.1", "50:28.1", "50:28.1", "50:28.2", "50:28.2", "50:28.2", "50:28.3", "50:28.3", "50:28.3", "50:28.4", "50:28.4", "50:28.4", "50:28.5", "50:28.5", "50:28.5", "50:28.6", "50:28.6", "50:28.6", "50:28.7", "50:28.7", "50:28.7", "50:28.8", "50:28.8", "50:28.8", "50:28.9", "50:28.9", "50:28.9", "50:29.0", "50:29.0", "50:29.0", "50:29.1", "50:29.1", "50:29.1", "50:29.2", "50:29.2", "50:29.2", "50:29.3", "50:29.3", "50:29.3", "50:29.4", "50:29.4", "50:29.4", "50:29.5", "50:29.5", "50:29.5", "50:29.6", "50:29.6", "50:29.6", "50:29.7", "50:29.7", "50:29.7", "50:29.8", "50:29.8", "50:29.8", "50:29.9", "50:29.9", "50:29.9", "50:30.0", "50:30.0", "50:30.0", "50:30.1", "50:30.1", "50:30.1", "50:30.2", "50:30.2", "50:30.2", "50:30.3", "50:30.3", "50:30.3", "50:30.4", "50:30.4", "50:30.4", "50:30.5", "50:30.5", "50:30.5", "50:30.6", "50:30.6", "50:30.6", "50:30.7", "50:30.7", "50:30.7", "50:30.8", "50:30.8", "50:30.8", "50:30.9", "50:30.9", "50:30.9", "50:31.0", "50:31.0", "50:31.0", "50:31.1", "50:31.1", "50:31.1", "50:31.2", "50:31.2", "50:31.2", "50:31.3", "50:31.3", "50:31.3", "50:31.4", "50:31.4", "50:31.4", "50:31.5", "50:31.5", "50:31.5", "50:31.6", "50:31.6", "50:31.6", "50:31.7", "50:31.7", "50:31.7", "50:31.8", "50:31.8", "50:31.8", "50:31.9", "50:31.9", "50:31.9", "50:32.0", "50:32.0", "50:32.0", "50:32.1", "50:32.1", "50:32.1", "50:32.2", "50:32.2", "50:32.2", "50:32.3", "50:32.3", "50:32.3", "50:32.4", "50:32.4", "50:32.4", "50:32.5", "50:32.5", "50:32.5", "50:32.6", "50:32.6", "50:32.6", "50:32.7", "50:32.7", "50:32.7", "50:32.8", "50:32.8", "50:32.8", "50:32.9", "50:32.9", "50:32.9", "50:33.0", "50:33.0", "50:33.0", "50:33.1", "50:33.1", "50:33.1", "50:33.2", "50:33.2", "50:33.2", "50:33.3", "50:33.3", "50:33.3", "50:33.4", "50:33.4", "50:33.4", "50:33.5", "50:33.5", "50:33.5", "50:33.6", "50:33.6", "50:33.6", "50:33.7", "50:33.7", "50:33.7", "50:33.8", "50:33.8", "50:33.8", "50:33.9", "50:33.9", "50:33.9", "50:34.0", "50:34.0", "50:34.0", "50:34.1", "50:34.1", "50:34.1", "50:34.2", "50:34.2", "50:34.2", "50:34.3", "50:34.3", "50:34.3", "50:34.4", "50:34.4", "50:34.4", "50:34.5", "50:34.5", "50:34.5", "50:34.6", "50:34.6", "50:34.6", "50:34.7", "50:34.7", "50:34.7", "50:34.8", "50:34.8", "50:34.8", "50:34.9", "50:34.9", "50:34.9", "50:35.0", "50:35.0", "50:35.0", "50:35.1", "50:35.1", "50:35.1", "50:35.2", "50:35.2", "50:35.2", "50:35.3", "50:35.3", "50:35.3", "50:35.4", "50:35.4", "50:35.4", "50:35.5", "50:35.5", "50:35.5", "50:35.6", "50:35.6", "50:35.6", "50:35.7", "50:35.7", "50:35.7", "50:35.8", "50:35.8", "50:35.8", "50:35.9", "50:35.9", "50:35.9", "50:36.0", "50:36.0", "50:36.0", "50:36.1", "50:36.1", "50:36.1", "50:36.2", "50:36.2", "50:36.2", "50:36.3", "50:36.3", "50:36.3", "50:36.4", "50:36.4", "50:36.4", "50:36.5", "50:36.5", "50:36.5", "50:36.6", "50:36.6", "50:36.6", "50:36.7", "50:36.7", "50:36.7", "50:36.8", "50:36.8", "50:36.8", "50:36.9", "50:36.9", "50:36.9", "50:37.0", "50:37.0", "50:37.0", "50:37.1", "50:37.1", "50:37.1", "50:37.2", "50:37.2", "50:37.2", "50:37.3", "50:37.3", "50:37.3", "50:37.4", "50:37.4", "50:37.4", "50:37.5", "50:37.5", "50:37.5", "50:37.6", "50:37.6", "50:37.6", "50:37.7", "50:37.7", "50:37.7", "50:37.8", "50:37.8", "50:37.8", "50:37.9", "50:37.9", "50:37.9", "50:38.0", "50:38.0", "50:38.0", "50:38.1", "50:38.1", "50:38.1", "50:38.2", "50:38.2", "50:38.2", "50:38.3", "50:38.3", "50:38.3", "50:38.4", "50:38.4", "50:38.4", "50:38.5", "50:38.5", "50:38.5", "50:38.6", "50:38.6", "50:38.6", "50:38.7", "50:38.7", "50:38.7", "50:38.8", "50:38.8", "50:38.8", "50:38.9", "50:38.9", "50:38.9", "50:39.0", "50:39.0", "50:39.0", "50:39.1", "50:39.1", "50:39.1", "50:39.2", "50:39.2", "50:39.2", "50:39.3", "50:39.3", "50:39.3", "50:39.4", "50:39.4", "50:39.4", "50:39.5", "50:39.5", "50:39.5", "50:39.6", "50:39.6", "50:39.6", "50:39.7", "50:39.7", "50:39.7", "50:39.8", "50:39.8", "50:39.8", "50:39.9", "50:39.9", "50:39.9", "50:40.0", "50:40.0", "50:40.0", "50:40.1", "50:40.1", "50:40.1", "50:40.2", "50:40.2", "50:40.2", "50:40.3", "50:40.3", "50:40.3", "50:40.4", "50:40.4", "50:40.4", "50:40.5", "50:40.5", "50:40.5", "50:40.6", "50:40.6", "50:40.6", "50:40.7", "50:40.7", "50:40.7", "50:40.8", "50:40.8", "50:40.8", "50:40.9", "50:40.9", "50:40.9", "50:41.0", "50:41.0", "50:41.0", "50:41.1", "50:41.1", "50:41.1", "50:41.2", "50:41.2", "50:41.2", "50:41.3", "50:41.3", "50:41.3", "50:41.4", "50:41.4", "50:41.4", "50:41.5", "50:41.5", "50:41.5", "50:41.6", "50:41.6", "50:41.6", "50:41.7", "50:41.7", "50:41.7", "50:41.8", "50:41.8", "50:41.8", "50:41.9", "50:41.9", "50:41.9", "50:42.0", "50:42.0", "50:42.0", "50:42.1", "50:42.1", "50:42.1", "50:42.2", "50:42.2", "50:42.2", "50:42.3", "50:42.3", "50:42.3", "50:42.4", "50:42.4", "50:42.4", "50:42.5", "50:42.5", "50:42.5", "50:42.6", "50:42.6", "50:42.6", "50:42.7", "50:42.7", "50:42.7", "50:42.8", "50:42.8", "50:42.8", "50:42.9", "50:42.9", "50:42.9", "50:43.0", "50:43.0", "50:43.0", "50:43.1", "50:43.1", "50:43.1", "50:43.2", "50:43.2", "50:43.2", "50:43.3", "50:43.3", "50:43.3", "50:43.4", "50:43.4", "50:43.4", "50:43.5", "50:43.5", "50:43.5", "50:43.6", "50:43.6", "50:43.6", "50:43.7", "50:43.7", "50:43.7", "50:43.8", "50:43.8", "50:43.8", "50:43.9", "50:43.9", "50:43.9", "50:44.0", "50:44.0", "50:44.0", "50:44.1", "50:44.1", "50:44.1", "50:44.2", "50:44.2", "50:44.2", "50:44.3", "50:44.3", "50:44.3", "50:44.4", "50:44.4", "50:44.4", "50:44.5", "50:44.5", "50:44.5", "50:44.6", "50:44.6", "50:44.6", "50:44.7", "50:44.7", "50:44.7", "50:44.8", "50:44.8", "50:44.8", "50:44.9", "50:44.9", "50:44.9", "50:45.0", "50:45.0", "50:45.0", "50:45.1", "50:45.1", "50:45.1", "50:45.2", "50:45.2", "50:45.2", "50:45.3", "50:45.3", "50:45.3", "50:45.4", "50:45.4", "50:45.4", "50:45.5", "50:45.5", "50:45.5", "50:45.6", "50:45.6", "50:45.6", "50:45.7", "50:45.7", "50:45.7", "50:45.8", "50:45.8", "50:45.8", "50:45.9", "50:45.9", "50:45.9", "50:46.0", "50:46.0", "50:46.0", "50:46.1", "50:46.1", "50:46.1", "50:46.2", "50:46.2", "50:46.2", "50:46.3", "50:46.3", "50:46.3", "50:46.4", "50:46.4", "50:46.4", "50:46.5", "50:46.5", "50:46.5", "50:46.6", "50:46.6", "50:46.6", "50:46.7", "50:46.7", "50:46.7", "50:46.8", "50:46.8", "50:46.8", "50:46.9", "50:46.9", "50:46.9", "50:47.0", "50:47.0", "50:47.0", "50:47.1", "50:47.1", "50:47.1", "50:47.2", "50:47.2", "50:47.2", "50:47.3", "50:47.3", "50:47.3", "50:47.4", "50:47.4", "50:47.4", "50:47.5", "50:47.5", "50:47.5", "50:47.6", "50:47.6", "50:47.6", "50:47.7", "50:47.7", "50:47.7", "50:47.8", "50:47.8", "50:47.8", "50:47.9", "50:47.9", "50:47.9", "50:48.0", "50:48.0", "50:48.0", "50:48.1", "50:48.1", "50:48.1", "50:48.2", "50:48.2", "50:48.2", "50:48.3", "50:48.3", "50:48.3", "50:48.4", "50:48.4", "50:48.4", "50:48.5", "50:48.5", "50:48.5", "50:48.6", "50:48.6", "50:48.6", "50:48.7", "50:48.7", "50:48.7", "50:48.8", "50:48.8", "50:48.8", "50:48.9", "50:48.9", "50:48.9", "50:49.0", "50:49.0", "50:49.0", "50:49.1", "50:49.1", "50:49.1", "50:49.2", "50:49.2", "50:49.2", "50:49.3", "50:49.3", "50:49.3", "50:49.4", "50:49.4", "50:49.4", "50:49.5", "50:49.5", "50:49.5", "50:49.6", "50:49.6", "50:49.6", "50:49.7", "50:49.7", "50:49.7", "50:49.8", "50:49.8", "50:49.8", "50:49.9", "50:49.9", "50:49.9", "50:50.0", "50:50.0", "50:50.0", "50:50.1", "50:50.1", "50:50.1", "50:50.2", "50:50.2", "50:50.2", "50:50.3", "50:50.3", "50:50.3", "50:50.4", "50:50.4", "50:50.4", "50:50.5", "50:50.5", "50:50.5", "50:50.6", "50:50.6", "50:50.6", "50:50.7", "50:50.7", "50:50.7", "50:50.8", "50:50.8", "50:50.8", "50:50.9", "50:50.9", "50:50.9", "50:51.0", "50:51.0", "50:51.0", "50:51.1", "50:51.1", "50:51.1", "50:51.2", "50:51.2", "50:51.2", "50:51.3", "50:51.3", "50:51.3", "50:51.4", "50:51.4", "50:51.4", "50:51.5", "50:51.5", "50:51.5", "50:51.6", "50:51.6", "50:51.6", "50:51.7", "50:51.7", "50:51.7", "50:51.8", "50:51.8", "50:51.8", "50:51.9", "50:51.9", "50:51.9", "50:52.0", "50:52.0", "50:52.0", "50:52.1", "50:52.1", "50:52.1", "50:52.2", "50:52.2", "50:52.2", "50:52.3", "50:52.3", "50:52.3", "50:52.4", "50:52.4", "50:52.4", "50:52.5", "50:52.5", "50:52.5", "50:52.6", "50:52.6", "50:52.6", "50:52.7", "50:52.7", "50:52.7", "50:52.8", "50:52.8", "50:52.8", "50:52.9", "50:52.9", "50:52.9", "50:53.0", "50:53.0", "50:53.0", "50:53.1", "50:53.1", "50:53.1", "50:53.2", "50:53.2", "50:53.2", "50:53.3", "50:53.3", "50:53.3", "50:53.4", "50:53.4", "50:53.4", "50:53.5", "50:53.5", "50:53.5", "50:53.6", "50:53.6", "50:53.6", "50:53.7", "50:53.7", "50:53.7", "50:53.8", "50:53.8", "50:53.8", "50:53.9", "50:53.9", "50:53.9", "50:54.0", "50:54.0", "50:54.0", "50:54.1", "50:54.1", "50:54.1", "50:54.2", "50:54.2", "50:54.2", "50:54.3", "50:54.3", "50:54.3", "50:54.4", "50:54.4", "50:54.4", "50:54.5", "50:54.5", "50:54.5", "50:54.6", "50:54.6", "50:54.6", "50:54.7", "50:54.7", "50:54.7", "50:54.8", "50:54.8", "50:54.8", "50:54.9", "50:54.9", "50:54.9", "50:55.0", "50:55.0", "50:55.0", "50:55.1", "50:55.1", "50:55.1", "50:55.2", "50:55.2", "50:55.2", "50:55.3", "50:55.3", "50:55.3", "50:55.4", "50:55.4", "50:55.4", "50:55.5", "50:55.5", "50:55.5", "50:55.6", "50:55.6", "50:55.6", "50:55.7", "50:55.7", "50:55.7", "50:55.8", "50:55.8", "50:55.8", "50:55.9", "50:55.9", "50:55.9", "50:56.0", "50:56.0", "50:56.0", "50:56.1", "50:56.1", "50:56.1", "50:56.2", "50:56.2", "50:56.2", "50:56.3", "50:56.3", "50:56.3", "50:56.4", "50:56.4", "50:56.4", "50:56.5", "50:56.5", "50:56.5", "50:56.6", "50:56.6", "50:56.6", "50:56.7", "50:56.7", "50:56.7", "50:56.8", "50:56.8", "50:56.8", "50:56.9", "50:56.9", "50:56.9", "50:57.0", "50:57.0", "50:57.0", "50:57.1", "50:57.1", "50:57.1", "50:57.2", "50:57.2", "50:57.2", "50:57.3", "50:57.3", "50:57.3", "50:57.4", "50:57.4", "50:57.4", "50:57.5", "50:57.5", "50:57.5", "50:57.6", "50:57.6", "50:57.6", "50:57.7", "50:57.7", "50:57.7", "50:57.8", "50:57.8", "50:57.8", "50:57.9", "50:57.9", "50:57.9", "50:58.0", "50:58.0", "50:58.0", "50:58.1", "50:58.1", "50:58.1", "50:58.2", "50:58.2", "50:58.2", "50:58.3", "50:58.3", "50:58.3", "50:58.4", "50:58.4", "50:58.4", "50:58.5", "50:58.5", "50:58.5", "50:58.6", "50:58.6", "50:58.6", "50:58.7", "50:58.7", "50:58.7", "50:58.8", "50:58.8", "50:58.8", "50:58.9", "50:58.9", "50:58.9", "50:59.0", "50:59.0", "50:59.0", "50:59.1", "50:59.1", "50:59.1", "50:59.2", "50:59.2", "50:59.2", "50:59.3", "50:59.3", "50:59.3", "50:59.4", "50:59.4", "50:59.4", "50:59.5", "50:59.5", "50:59.5", "50:59.6", "50:59.6", "50:59.6", "50:59.7", "50:59.7", "50:59.7", "50:59.8", "50:59.8", "50:59.8", "50:59.9", "50:59.9", "50:59.9", "51:00.0"]
  in  "OK Button":bool
